vi "Frontend FPP_vdp_Ian_modified v3.0.vi"() -> ()   [LabVIEW 2016]
panel:
  in  "Gate 2":T1={"Gate Start"=0.0, "Gate Stop"=2.0, "Gate Step (linear only)"=1.0, "Gate Compliance"=0.0001, "Gate PComp"=0.0, "Range mode"=0, "Range"=6} {"Range" max=11 scale=0.0..11.0; "Range mode" items=["Auto", "Limited", "Fixed"]; "Gate PComp" format="%^.2e"; "Gate Compliance" format="%^.2e"; "Gate Step (linear only)" format="%^.4e"; "Gate Stop" format="%^.4e"; "Gate Start" format="%^.4e"}
  in  "Drain":T2={"Drain Start"=0.0, "Drain Stop"=2.0, "Drain Compliance"=0.0001, "Drain Step"=1.0, "Drain PComp"=0.0, "Range mode"=0, "Range"=6} {"Range" max=11 scale=0.0..11.0; "Range mode" items=["Auto", "Limited", "Fixed"]; "Drain PComp" format="%^.2e"; "Drain Step" format="%^.4e"; "Drain Compliance" format="%^.2e"; "Drain Stop" format="%^.4e"; "Drain Start" format="%^.4e"}
  in  "Gate":T3={"Gate Start"=0.0, "Gate Stop"=2.0, "Gate Step"=1.0, "Gate Compliance"=0.0001, "Gate PComp"=0.0, "Range mode"=0, "Range"=6} {"Range" max=11 scale=0.0..11.0; "Range mode" items=["Auto", "Limited", "Fixed"]; "Gate PComp" format="%^.2e"; "Gate Compliance" format="%^.2e"; "Gate Step" format="%^.4e"; "Gate Stop" format="%^.4e"; "Gate Start" format="%^.4e"}
  in  "Drain 2":T4={"Drain Start"=0.0, "Drain Stop"=2.0, "Drain Compliance"=0.0001, "Drain Step (linear only)"=1.0, "Drain PComp"=0.0, "Range mode"=0, "Range"=6} {"Range" max=11 scale=0.0..11.0; "Range mode" items=["Auto", "Limited", "Fixed"]; "Drain PComp" format="%^.2e"; "Drain Step (linear only)" format="%^.4e"; "Drain Compliance" format="%^.2e"; "Drain Stop" format="%^.4e"; "Drain Start" format="%^.4e"}
  in  "Timings":T5={"integration time"=0, "Short/Long integration time"=0.00064, "hold time (sec)"=0.0, "delay time (sec)"=0.0, "Step Time (0 disables)"=0.0, "sweep method"=0, "Pulse period"=0.005, "Base voltage"=0.0, "Pulse width"=0.0005} {"Pulse width" min=0.0005 max=0.1 step=0.0001 format="%.4f"; "Base voltage" format="%^.4e"; "Pulse period" min=0.005 max=1.0 step=0.0001 format="%.4f"; "sweep method" items=["Continuous", "Pulsed"]; "Step Time (0 disables)" format="%.2f"; "delay time (sec)" format="%.4f"; "hold time (sec)" format="%.4f"; "Short/Long integration time" format="%^.0e"; "integration time" scale=0.0..2.0}
  in  "Panel controls":T6={"Emergency Stop"=refnum, "OutputGraph Max"=1e-05, "Text/Graph (text=false)"=FALSE} {"OutputGraph Max" format="%.2e"}
  in  "Panel Controls":T7={"Emergency Stop"=refnum, "TransGraph Max"=1e-05, "Text/Graph (text=false)"=FALSE} {"TransGraph Max" format="%.2e"}
  in  "Tab Control":enum32{"Characteristics", "Other parameters"}(tab)
  in  "FPP - Source":u32(ring)=6 items=["SMU1  ", "SMU2  ", "SMU3  ", "SMU4  ", "SMU5  ", "SMU6  ", "VSU1  ", "VSU2  "]
  in  "FPP - Drain":u32(ring)=1 items=["SMU1  ", "SMU2  ", "SMU3  ", "SMU4  ", "SMU5  ", "SMU6  ", "VSU1  ", "VSU2  "]
  in  "FPP - Gate":u32(ring)=2 items=["SMU1  ", "SMU2  ", "SMU3  ", "SMU4  ", "SMU5  ", "SMU6  ", "VSU1  ", "VSU2  "]
  in  "FPP - Probe 1":u32(ring) items=["SMU1  ", "SMU2  ", "SMU3  ", "SMU4  ", "SMU5  ", "SMU6  ", "VSU1  ", "VSU2  "]
  in  "FPP - Probe 2":u32(ring)=3 items=["SMU1  ", "SMU2  ", "SMU3  ", "SMU4  ", "SMU5  ", "SMU6  ", "VSU1  ", "VSU2  "]
  in  "Van der Pauw":bool
  out "XY Graph 2":cluster{"Y data in":dbl[], "X data in":dbl[]}[](graph)
  in  "Integration time (long)":dbl=0.32 min=0.04 max=2.0 step=0.02 format="%.2f"
  in  "Integration time (short)":dbl=0.00064 min=8e-05 max=0.00192 step=8e-05 format="%^.0e"
  in  "Drain Range":u8(slide)=6 max=11 scale=0.0..11.0
  in  "Drain Range mode":u16(ring) items=["Auto", "Limited", "Fixed"]
  in  "Gate Range":u8(slide)=6 max=11 scale=0.0..11.0
  in  "Gate Range mode":u16(ring) items=["Auto", "Limited", "Fixed"]
  in  "Sampling mode":u32(slide) scale=0.0..4.0
  in  "Number of Samples":i32=500 min=0 step=1
  in  "Time":dbl=240.0 min=0.0 format="%.2f"
  in  "Drain":dbl=-10.0 min=-100.0 max=100.0 format="%.2f"
  in  "Gate":dbl=-60.0 min=-100.0 max=100.0 format="%.2f"
  in  "sweep method":u16(ring) items=["Continuous", "Pulsed"]
  out "Id":dbl format="%.2e"
  out "Ig":dbl format="%.2e"
  in  "Sweep Start":bool caption="Sweep start"
  in  "Interrupt run":bool
  in  "Running":bool=TRUE
  out "Path":path
  in  "integration time":u32(slide)=1 max=2 step=1 scale=0.0..2.0
  in  "sweep mode":u16(ring)=1 items=["Single", "Double"]
  in  "Transfer Start":bool
  in  "Output Start":bool
  in  "Drain: Step":dbl=-0.1 min=-100.0 max=100.0 format="%.2f"
  in  "Drain: Stop":dbl=-1.0 min=-100.0 max=100.0 format="%.2f"
  in  "Drain:Start":dbl=1.0 min=-100.0 max=100.0 format="%.2f"
  in  "Gate: Step":dbl min=-100.0 max=100.0 format="%.2f"
  in  "Gate: Stop":dbl min=-100.0 max=100.0 format="%.2f"
  in  "Gate: Start":dbl min=-100.0 max=100.0 format="%.2f"
  out "XY Graph":cluster{"Y data in":dbl[], "X data in":dbl[]}[](graph)
  in  "Drain: Compliance":dbl=0.001 min=1e-12 max=0.02 format="%.8f"
  in  "Gate: Compliance":dbl=0.001 min=1e-12 max=0.02 format="%.8f"
  in  "Drain: Step":dbl=-5.0 min=-100.0 max=100.0 format="%.2f"
  in  "Drain: Stop":dbl=-10.0 min=-100.0 max=100.0 format="%.2f"
  in  "Drain:Start":dbl=-5.0 min=-100.0 max=100.0 format="%.2f"
  in  "Gate: Step":dbl=-1.0 min=-100.0 max=100.0 format="%.2f"
  in  "Gate: Stop":dbl=-60.0 min=-100.0 max=100.0 format="%.2f"
  in  "Gate: Start":dbl=10.0 min=-100.0 max=100.0 format="%.2f"
  out "Vp_2":dbl format="%.2e"
  out "Vp_1":dbl format="%.2e"
  out "Delta V":dbl format="%.2e"
  out "Conductivity (S/cm)":dbl format="%.2e"
  in  "Thickness (m)":dbl=4e-08 min=1e-09 max=100.0 format="%.2e"
  in  "Hall Bar Channel Length  (L in m)":dbl=2e-05 format="%#_13g"
  in  "Hall Bar Channel Width (W in m)":dbl=4e-05 format="%#_13g"
  in  "Pulse width":dbl=0.0005 min=0.0005 max=0.1 step=0.0001 format="%.4f"
  in  "Base voltage":dbl min=-100.0 max=100.0 format="%.2f"
  in  "Pulse period":dbl=0.005 min=0.005 max=1.0 step=0.0001 format="%.4f"
  in  "Drain Power Compliance":dbl min=0.0 max=1.0 format="%.2f"
  in  "Gate Power\nCompliance":dbl min=0.0 max=1.0 format="%.2f"
  in  "OutputGraph Max":dbl=1e-05 format="%.2e"
  in  "TransGraph Max":dbl=1e-05 format="%.2e"
  in  "SPA Display":bool
  in  "Step delay /s":dbl min=0.0 max=1.0 format="%.2f"
  in  "hold time /s":dbl min=0.0 max=655.35 step=0.01 format="%.2f"
  in  "delay time /s":dbl min=0.0 max=65.535 step=0.0001 format="%.2f"
  in  "Decimal places in header":i8=1
  out "error out":errorcluster
  # "Transfer Characteristics"
  # "Stress Measurements"
  # "V"
  # "V"
  # "V"
  # "Gate"
  # "V"
  # "V"
  # "V"
  # "V"
  # "Drain"
  # "V"
  # "Output Characteristics"
  # "s"
  # "V"
  # "V"
  # "V"
  # "Gate"
  # "V"
  # "V"
  # "Drain"
  # "V"
  # "For Four Point Probe measurements ONLY!"
  # "A"
  # "A"
  # "Vp1"
  # "Vp2"
  # "Pulsed mode settings"
  # "NOTE - THIS OVERRIDES THE COMPLIANCE VALUES!"
  # "A"
  # "A"
  # "Enter max power in Watts (max 1W)"
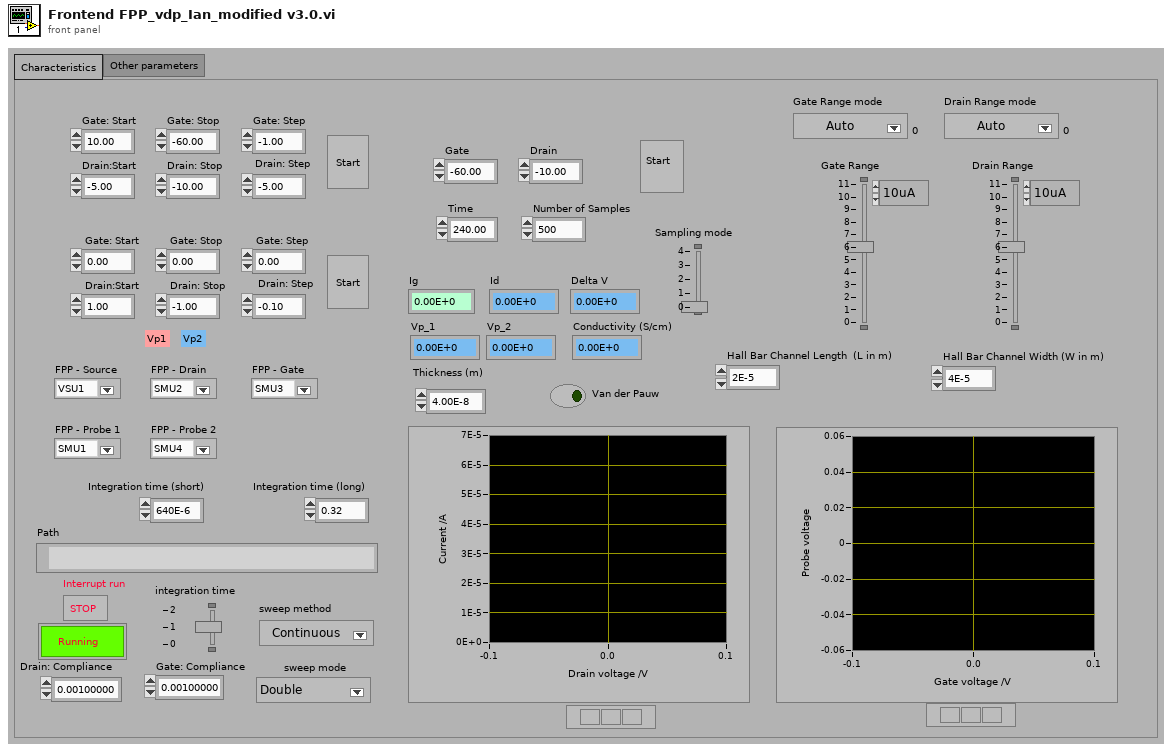
[diagram p1: front panel]
types:
  T1 = cluster{"Gate Start":dbl, "Gate Stop":dbl, "Gate Step (linear only)":dbl, "Gate Compliance":dbl, "Gate PComp":dbl, "Range mode":u16, "Range":u8}
  T2 = cluster{"Drain Start":dbl, "Drain Stop":dbl, "Drain Compliance":dbl, "Drain Step":dbl, "Drain PComp":dbl, "Range mode":u16, "Range":u8}
  T3 = cluster{"Gate Start":dbl, "Gate Stop":dbl, "Gate Step":dbl, "Gate Compliance":dbl, "Gate PComp":dbl, "Range mode":u16, "Range":u8}
  T4 = cluster{"Drain Start":dbl, "Drain Stop":dbl, "Drain Compliance":dbl, "Drain Step (linear only)":dbl, "Drain PComp":dbl, "Range mode":u16, "Range":u8}
  T5 = cluster{"integration time":u32, "Short/Long integration time":dbl, "hold time (sec)":dbl, "delay time (sec)":dbl, "Step Time (0 disables)":dbl, "sweep method":u16, "Pulse period":dbl, "Base voltage":dbl, "Pulse width":dbl}
  T6 = cluster{"Emergency Stop":refnum<vi>, "OutputGraph Max":dbl, "Text/Graph (text=false)":bool}
  T7 = cluster{"Emergency Stop":refnum<vi>, "TransGraph Max":dbl, "Text/Graph (text=false)":bool}
  T8 = cluster{"V2 Start":dbl, "V2 Step":dbl, "Number of points":i32}
  T9 = enum16{"open", "replace", "create", "open or create", "replace or create", "replace or create with confirmation"}
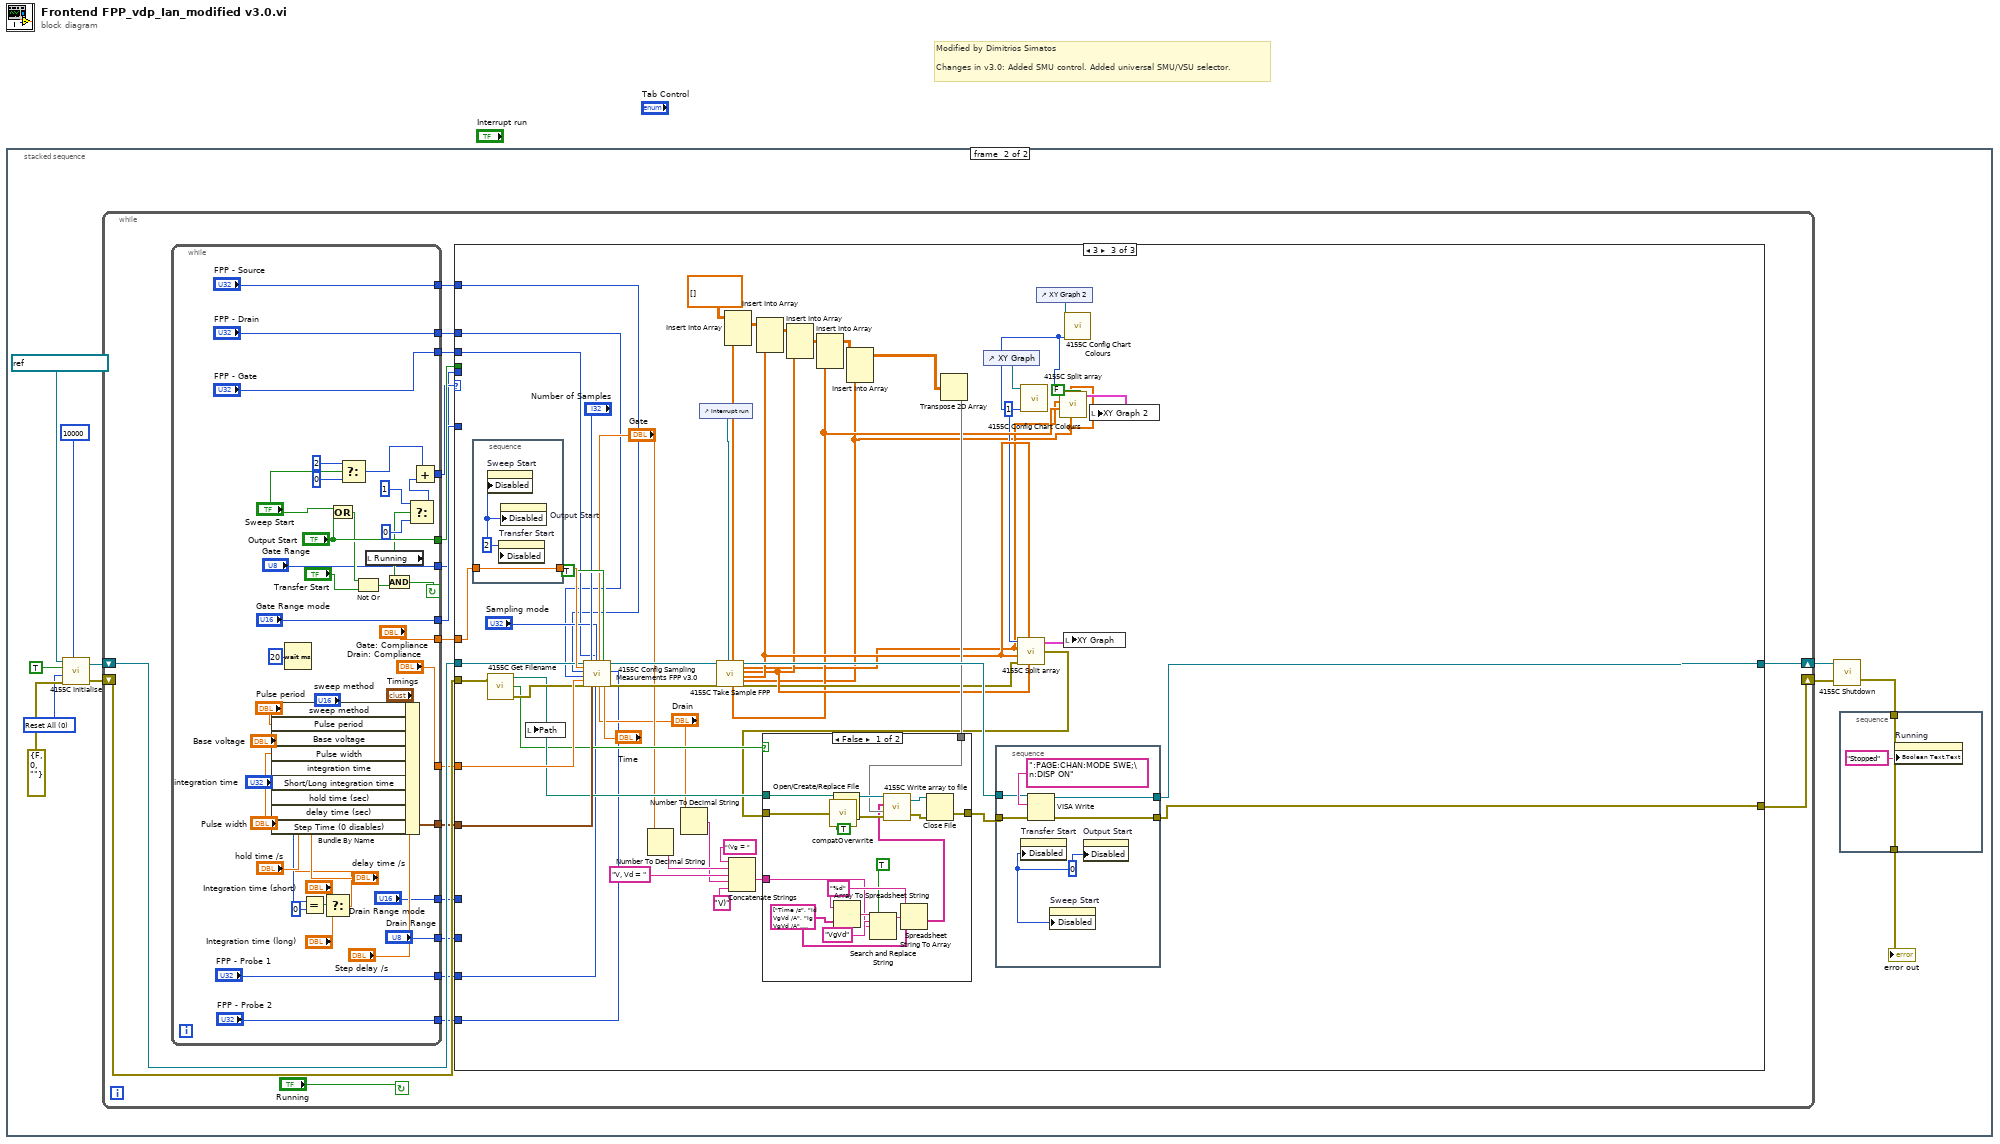
[diagram p0: block diagram]
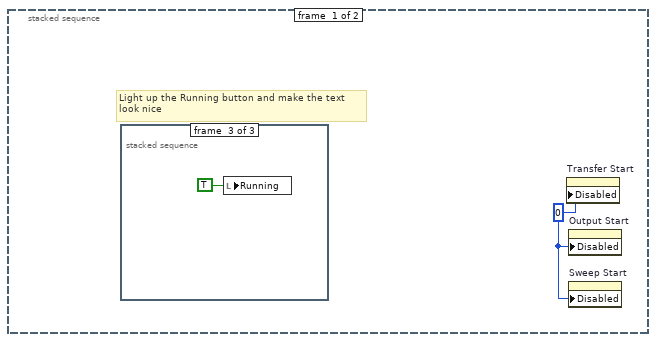
[diagram p2: hidden frame]
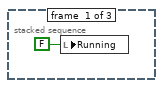
[diagram p3: hidden frame]
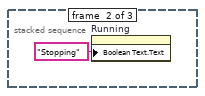
[diagram p4: hidden frame]
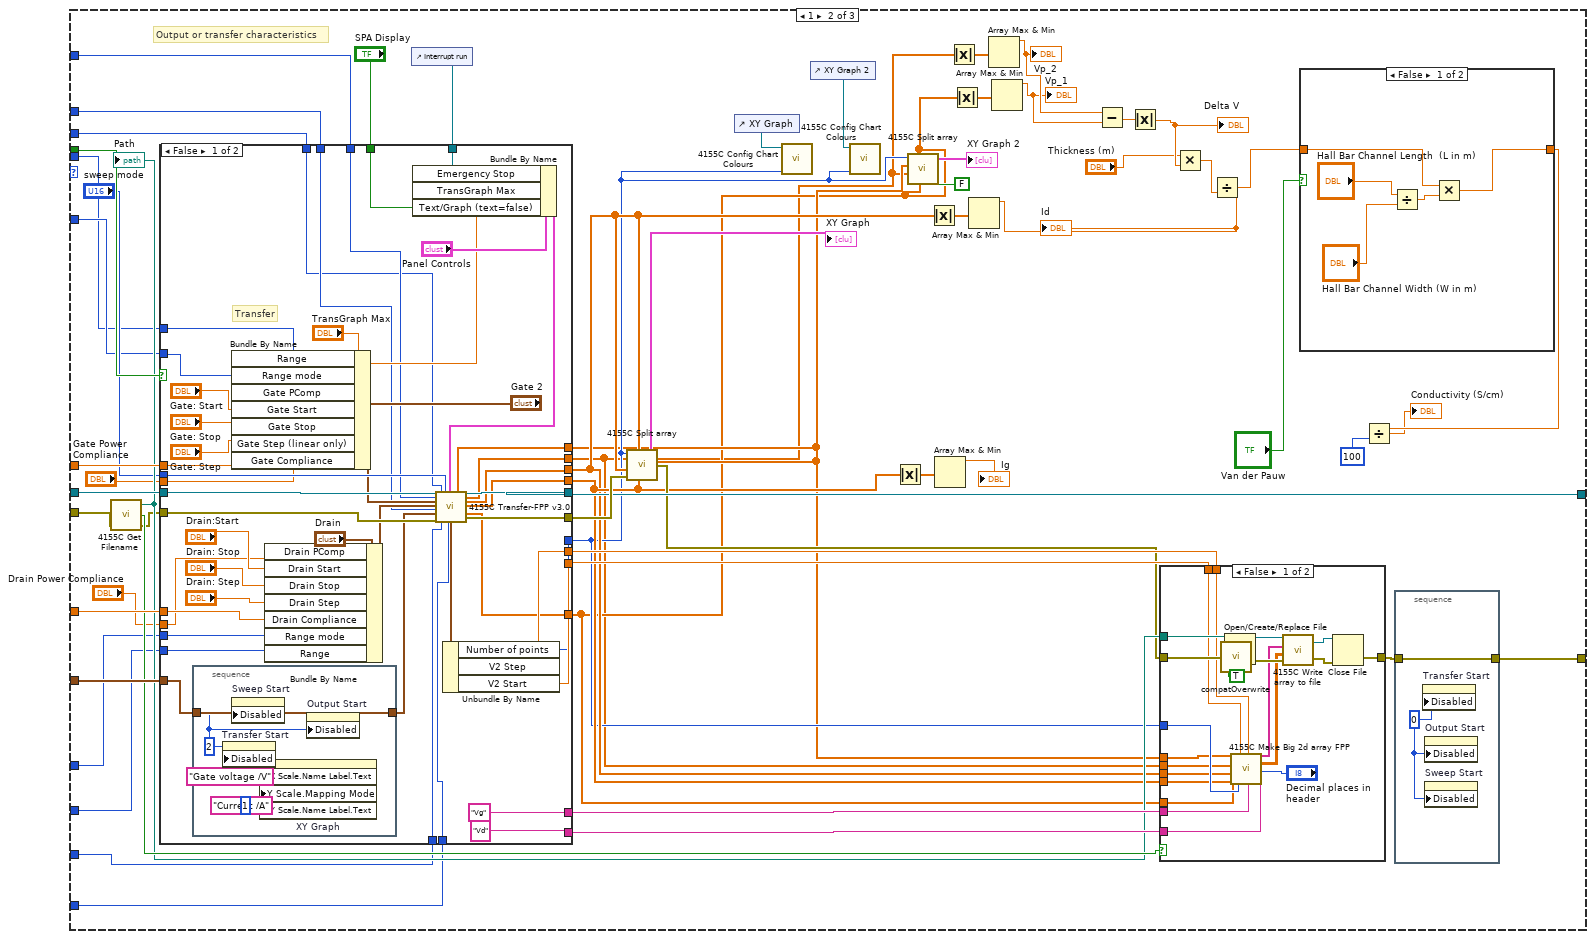
[diagram p6: hidden frame]
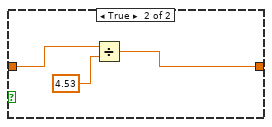
[diagram p7: hidden frame]
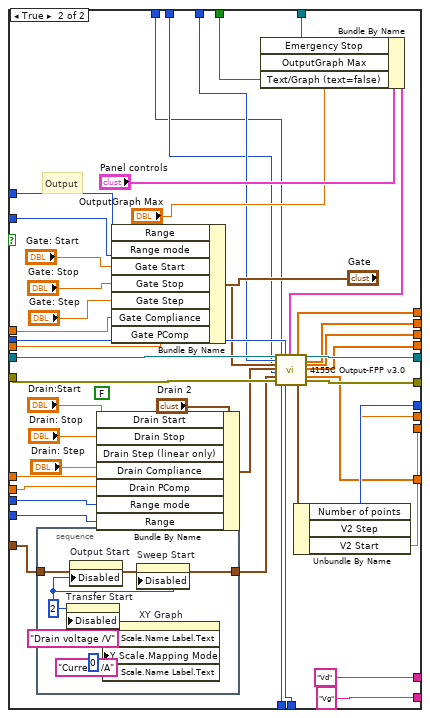
[diagram p9: hidden frame]
diagram:
  # "Modified by Dimitrios Simatos\n\nChanges in v3.0: Added SMU control. Added universal SMU/VSU selector."
  n1 = stacked-sequence {
    frame #0 {
      w1 = u8 0 ("Disabled")
      # "Light up the Running button and make the text\nlook nice"
      n2 = stacked-sequence {
        frame #0 {
          n3 = local write "Running"(FALSE ("Running")) -> ()
        }
        frame #1 {
          n4 = property on="Running" class="Bool (strict)"("Boolean Text.Text"="Stopping") -> ()  [unwired: 2 in, 2 out]
        }
        frame #2 {
          (unwired) FALSE ("Running")
          n5 = local write "Running"(TRUE ("Running")) -> ()
        }
      }
      n6 = property on="Transfer Start" class="Bool (strict)"("Disabled"=w1) -> ()  [unwired: 2 in, 2 out]
      n7 = property on="Output Start" class="Bool (strict)"("Disabled"=w1) -> ()  [unwired: 2 in, 2 out]
      n8 = property on="Sweep Start" class="Bool (strict)"("Disabled"=w1) -> ()  [unwired: 2 in, 2 out]
    }
    frame #1 {
      w11 = u16 0 items=["Reset All", "Partial reset"] ("Type of reset")
      n9 = call "4155C Initialise.vi"("VISA resource name in"=refnum<visa-resource-name> "GPIB0::14::INSTR", "Reset"=TRUE, "Type of reset"=w11, "error in (no error)"=errorcluster {"status"=FALSE, "code"=0, "source"=""}, "VISA Timeout Value"=u32 10000) -> ("VISA Resource Name out"=w10:refnum<visa-resource-name>, "error out"=w9:errorcluster)
      n10 = while {
        shift-left: w10 -> [w29]
        shift-right: [w31] -> w5
        shift-left: w9 -> [w30]
        shift-right: [w32] -> w6
        stop <- "Running" continue-if-true
        n11 = while {
          tunnel: ["Gate Range"] -> w21
          tunnel: ["Gate Range mode"] -> w22
          tunnel: ["Drain Range"] -> w23
          tunnel: ["Drain Range mode"] -> w24
          tunnel: ["Drain: Compliance"] -> w25
          tunnel: [w59] -> w26
          tunnel: ["Gate: Compliance"] -> w27
          tunnel: [w65] -> w28
          tunnel: ["Output Start"] -> w33
          tunnel: ["FPP - Probe 1"] -> w20
          tunnel: ["FPP - Probe 2"] -> w19
          tunnel: ["FPP - Gate"] -> w18
          tunnel: ["FPP - Drain"] -> w17
          tunnel: ["FPP - Source"] -> w16
          stop <- w74 continue-if-true
          n12 = Wait (ms)(milliseconds to wait=u32 20) -> ()  [unwired: 1 out]
          n13 = Equal?(x="integration time", y=u32 0) -> (x = y?=w56:bool)
          n14 = Select(t="Integration time (short)", s=w56, f="Integration time (long)") -> (s? t:f=w53:dbl)
          n15 = Bundle By Name(cluster="Timings", "sweep method"="sweep method", "Pulse period"="Pulse period", "Base voltage"="Base voltage", "Pulse width"="Pulse width", "integration time"="integration time", "Short/Long integration time"=w53, "hold time (sec)"="hold time /s", "delay time (sec)"="delay time /s", "Step Time (0 disables)"="Step delay /s") -> (w59:T5)
          n16 = Or(x="Sweep Start", y="Output Start") -> (x .or. y?=w71:bool)
          n17 = Select(t=i8 2, s="Sweep Start", f=i8 0) -> (s? t:f=w41:i8)
          n18 = Not Or(1:"Transfer Start", 2:w71) -> (0:w73:bool)
          n19 = local read "Running"() -> (w68:bool)
          n20 = And(x=w68, y=w73) -> (x .and. y?=w74:bool)
          n21 = Select(t=i8 1, s=w68, f=i8 0) -> (s? t:f=w64:i8)
          n22 = Add(x=w41, y=w64) -> (x+y=w65:i8)
        }
        n23 = case shown="3" w28 {
          tunnel: w33 -> [_ w137 _]
          tunnel: w26 -> [_ w136 w317]
          tunnel: w27 -> [_ w135 w325]
          tunnel: w25 -> [_ w134 w321]
          tunnel: [w77 w125 w323] -> w32
          tunnel: [w76 w128 w324] -> w31
          tunnel: w30 -> [w77 w119 w312]
          tunnel: w29 -> [w76 w127 w311]
          tunnel: w24 -> [_ w109 _]
          tunnel: w23 -> [_ w108 _]
          tunnel: w22 -> [_ w107 _]
          tunnel: w21 -> [_ w106 _]
          tunnel: w20 -> [_ w79 w277]
          tunnel: w19 -> [_ w78 w276]
          tunnel: w18 -> [_ w80 w275]
          tunnel: w17 -> [_ w81 w274]
          tunnel: w16 -> [_ w82 w273]
          frame 0, Default {
            # "Someone's deselected the running button so just shutdown..."
          }
          frame 1 {
            # "Output or transfer characteristics"
            n24 = call "4155C Get Filename.vi"("error in (no error)"=w119) -> ("error out"=w118:errorcluster, "cancelled"=w124:bool, "path"=w123:path)  [unwired: 2 in]
            "Path" <- w123
            n25 = control-ref of="Interrupt run"() -> (w120:refnum<vi>)
            n26 = case shown="False" w137 {
              tunnel: w127 -> [w202 w253]
              tunnel: w118 -> [w201 w252]
              tunnel: w136 -> [w205 w258]
              tunnel: w135 -> [w211 w265]
              tunnel: w134 -> [w216 w264]
              tunnel: "sweep mode" -> [w210 w263]
              tunnel: [w178 w231] -> w100
              tunnel: [w177 w230] -> w95
              tunnel: [w180 w229] -> w105
              tunnel: [w179 w228] -> w110
              tunnel: [w209 w262] -> w128
              tunnel: [w208 w261] -> w133
              tunnel: [w181 w234] -> w101
              tunnel: [w182 w233] -> w131
              tunnel: [w183 w232] -> w132
              tunnel: ["Vg" "Vd"] -> w130
              tunnel: ["Vd" "Vg"] -> w129
              tunnel: w120 -> [w199 w251]
              tunnel: "SPA Display" -> [w198 w249]
              tunnel: "Drain Power Compliance" -> [w194 w246]
              tunnel: "Gate Power\nCompliance" -> [w195 w245]
              tunnel: w109 -> [w186 w239]
              tunnel: w108 -> [w185 w238]
              tunnel: w107 -> [w187 w237]
              tunnel: w106 -> [w188 w236]
              tunnel: [w176 w227] -> w97
              tunnel: w82 -> [w175 w226]
              tunnel: w81 -> [w174 w225]
              tunnel: w80 -> [w173 w224]
              tunnel: w79 -> [w172 w223]
              tunnel: w78 -> [w171 w222]
              frame False {
                # "Transfer"
                n27 = stacked-sequence {
                  tunnel: w205 -> [w220]
                  tunnel: [w220] -> w193
                  frame #0 {
                    w218 = u8 2 ("Disabled")
                    n28 = property on="Transfer Start" class="Bool (strict)"("Disabled"=w218) -> ()  [unwired: 2 in, 2 out]
                    n29 = property on="Sweep Start" class="Bool (strict)"("Disabled"=w218) -> ()  [unwired: 2 in, 2 out]
                    n30 = property on="XY Graph" class="XYGraph (strict)"("X Scale.Name Label.Text"="Gate voltage /V", "Y Scale.Mapping Mode"=u8 1, "Y Scale.Name Label.Text"="Current /A") -> ()  [unwired: 2 in, 2 out]
                    n31 = property on="Output Start" class="Bool (strict)"("Disabled"=w218) -> ()  [unwired: 2 in, 2 out]
                  }
                }
                n32 = Bundle By Name(cluster="Gate 2", "Range"=w188, "Range mode"=w187, "Gate PComp"=w195, "Gate Start"="Gate: Start", "Gate Stop"="Gate: Stop", "Gate Step (linear only)"="Gate: Step", "Gate Compliance"=w211) -> (w189:T1)
                n33 = Bundle By Name(cluster="Drain", "Drain PComp"=w194, "Drain Start"="Drain:Start", "Drain Stop"="Drain: Stop", "Drain Step"="Drain: Step", "Drain Compliance"=w216, "Range mode"=w186, "Range"=w185) -> (w191:T2)
                n34 = Bundle By Name(cluster="Panel Controls", "Emergency Stop"=w199, "TransGraph Max"="TransGraph Max", "Text/Graph (text=false)"=w198) -> (w196:T7)
                n35 = call "4155C Transfer-FPP v3.0.vi"("VISA resource name in"=w202, "FPP - Source"=w175, "Gate"=w189, "Drain"=w191, "FPP - Drain"=w174, "Timings"=w193, "error in (no error)"=w201, "FPP - Gate"=w173, "FPP - Probe 1"=w172, "sweep mode"=w210, "FPP - Probe 2"=w171, "Panel Controls"=w196) -> ("VG"=w178:dbl[], "Outparams"=w184:T8, "VISA Resource Name out"=w209:refnum<visa-resource-name>, "Vprobe2"=w177:dbl[], "ID"=w180:dbl[], "IG"=w179:dbl[], "Vprobe1"=w176:dbl[], "error out"=w208:errorcluster)  [unwired: 8 in]
                n36 = Unbundle By Name(w184) -> ("Number of points"=w181:i32, "V2 Step"=w182:dbl, "V2 Start"=w183:dbl)
              }
              frame True {
                (unwired) FALSE ("Logarithmic")
                # "Output"
                n37 = stacked-sequence {
                  tunnel: w258 -> [w271]
                  tunnel: [w271] -> w244
                  frame #0 {
                    w269 = u8 2 ("Disabled")
                    n38 = property on="Transfer Start" class="Bool (strict)"("Disabled"=w269) -> ()  [unwired: 2 in, 2 out]
                    n39 = property on="Output Start" class="Bool (strict)"("Disabled"=w269) -> ()  [unwired: 2 in, 2 out]
                    n40 = property on="XY Graph" class="XYGraph (strict)"("X Scale.Name Label.Text"="Drain voltage /V", "Y Scale.Mapping Mode"=u8 0, "Y Scale.Name Label.Text"="Current /A") -> ()  [unwired: 2 in, 2 out]
                    n41 = property on="Sweep Start" class="Bool (strict)"("Disabled"=w269) -> ()  [unwired: 2 in, 2 out]
                  }
                }
                n42 = Bundle By Name(cluster="Drain 2", "Drain Start"="Drain:Start", "Drain Stop"="Drain: Stop", "Drain Step (linear only)"="Drain: Step", "Drain Compliance"=w264, "Drain PComp"=w246, "Range mode"=w239, "Range"=w238) -> (w242:T4)
                n43 = Bundle By Name(cluster="Gate", "Range"=w236, "Range mode"=w237, "Gate Start"="Gate: Start", "Gate Stop"="Gate: Stop", "Gate Step"="Gate: Step", "Gate Compliance"=w265, "Gate PComp"=w245) -> (w240:T3)
                n44 = Bundle By Name(cluster="Panel controls", "Emergency Stop"=w251, "OutputGraph Max"="OutputGraph Max", "Text/Graph (text=false)"=w249) -> (w247:T6)
                n45 = call "4155C Output-FPP v3.0.vi"("VISA resource name in"=w253, "FPP - Source"=w226, "Gate"=w240, "Drain"=w242, "FPP - Drain"=w225, "Timings"=w244, "error in (no error)"=w252, "FPP - Gate"=w224, "FPP - Probe 1"=w223, "sweep mode"=w263, "FPP - Probe 2"=w222, "Panel controls"=w247) -> ("VD"=w231:dbl[], "Outparams"=w235:T8, "VISA Resource Name out"=w262:refnum<visa-resource-name>, "Vprobe2"=w230:dbl[], "ID"=w229:dbl[], "IG"=w228:dbl[], "Vprobe1"=w227:dbl[], "error out"=w261:errorcluster)  [unwired: 8 in]
                n46 = Unbundle By Name(w235) -> ("Number of points"=w234:i32, "V2 Step"=w233:dbl, "V2 Start"=w232:dbl)
              }
            }
            n47 = call "4155C Split array.vi"("Number of VAR2 steps"=w101, "Y2 data in"=w105, "X data in"=w100, "Y1 data in"=w105, "Y3 data in"=w110, "error in (no error)"=w133) -> ("Array of clusters"=→"XY Graph":cluster{"Y data in":dbl[], "X data in":dbl[]}[], "error out"=w117:errorcluster)  [unwired: 1 in]
            n48 = control-ref of="XY Graph"() -> (w121:refnum<vi>)
            n49 = call "4155C Config Chart Colours.vi"("Numeric"=w101, "XY Graph 2"=w121) -> ()  [unwired: 6 in]
            n50 = control-ref of="XY Graph 2"() -> (w103:refnum<vi>)
            n51 = call "4155C Config Chart Colours.vi"("Numeric"=w101, "XY Graph 2"=w103) -> ()  [unwired: 6 in]
            n52 = Absolute Value(x=w110) -> (abs(x)=w112:dbl[])
            n53 = call "4155C Split array.vi"("Number of VAR2 steps"=w101, "Y2 data in"=w97, "X data in"=w100, "Y1 data in"=w95, "Y3 data in"=w97, "Absolute val?"=FALSE) -> ("Array of clusters"=→"XY Graph 2":cluster{"Y data in":dbl[], "X data in":dbl[]}[])  [unwired: 1 in, 1 out]
            n54 = Absolute Value(x=w105) -> (abs(x)=w111:dbl[])
            n55 = Array Max & Min(array=w112) -> (max value=→"Ig":dbl)  [unwired: 3 out]
            n56 = Absolute Value(x=w95) -> (abs(x)=w96:dbl[])
            n57 = Absolute Value(x=w97) -> (abs(x)=w98:dbl[])
            n58 = Array Max & Min(array=w111) -> (max value=w86:dbl)  [unwired: 3 out]
            "Id" <- w86
            n59 = Array Max & Min(array=w96) -> (max value=w94:dbl)  [unwired: 3 out]
            "Vp_2" <- w94
            n60 = Array Max & Min(array=w98) -> (max value=w93:dbl)  [unwired: 3 out]
            "Vp_1" <- w93
            n61 = Subtract(x=w94, y=w93) -> (x-y=w92:dbl)
            n62 = Absolute Value(x=w92) -> (abs(x)=w91:dbl)
            "Delta V" <- w91
            n63 = case shown="False" w124 {
              tunnel: w117 -> [w168 w170]
              tunnel: [w163 w170] -> w126
              tunnel: w123 -> [w167 _]
              tunnel: w101 -> [w161 _]
              tunnel: w105 -> [w151 _]
              tunnel: w100 -> [w153 _]
              tunnel: w95 -> [w152 _]
              tunnel: w110 -> [w150 _]
              tunnel: w132 -> [w155 _]
              tunnel: w131 -> [w156 _]
              tunnel: w130 -> [w160 _]
              tunnel: w129 -> [w159 _]
              tunnel: w97 -> [w149 _]
              frame False {
                n64 = call <vilib>:"compatOverwrite.vi"("overwrite (F)"=TRUE) -> ("overwrite?"=w148:T9)
                n65 = Open/Create/Replace File(file path (use dialog)=w167, error in=w168, operation (0:open)=w148) -> (refnum out=w165:refnum<file>, error out=w166:errorcluster)  [unwired: 3 in, 1 out]
                n66 = call "4155C Make Big 2d array FPP.vi"("1D Var1"=w153, "1d ID"=w151, "1d Vp2"=w152, "1d IG"=w150, "1d Vp1"=w149, "VAR2 START"=w155, "Number of VAR2 steps"=w161, "VAR2 STEP"=w156, "VAR1 Name"=w160, "Decimal places in header"="Decimal places in header", "VAR2 Name"=w159) -> ("Header array"=w157:string[], "Data array"=w158:dbl[][])  [unwired: 15 in]
                n67 = call "4155C Write array to file.vi"("Byte Stream File Refnum"=w165, "Header"=w157, "Data Array"=w158, "error in (no error)"=w166) -> ("dup refnum"=w162:refnum<file>, "error out"=w164:errorcluster)  [unwired: 1 in]
                n68 = Close File(refnum=w162, error in=w164) -> (error out=w163:errorcluster)  [unwired: 1 out]
              }
              frame True {
              }
            }
            n69 = Multiply(x="Thickness (m)", y=w91) -> (x*y=w87:dbl)
            n70 = Divide(x=w86, y=w87) -> (x/y=w88:dbl)
            n71 = case shown="False" "Van der Pauw" {
              tunnel: [w140 w144] -> w85
              tunnel: w88 -> [w141 w145]
              frame False {
                n72 = Divide(x="Hall Bar Channel Length  (L in m)", y="Hall Bar Channel Width (W in m)") -> (x/y=w142:dbl)
                n73 = Multiply(x=w141, y=w142) -> (x*y=w140:dbl)
              }
              frame True {
                n74 = Divide(x=w145, y=4.53) -> (x/y=w144:dbl)
              }
            }
            n75 = Divide(x=w85, y=100) -> (x/y=→"Conductivity (S/cm)":dbl)
            n76 = stacked-sequence {
              tunnel: w126 -> [w147]
              tunnel: [w147] -> w125
              frame #0 {
                w146 = u8 0 ("Disabled")
                n77 = property on="Transfer Start" class="Bool (strict)"("Disabled"=w146) -> ()  [unwired: 2 in, 2 out]
                n78 = property on="Output Start" class="Bool (strict)"("Disabled"=w146) -> ()  [unwired: 2 in, 2 out]
                n79 = property on="Sweep Start" class="Bool (strict)"("Disabled"=w146) -> ()  [unwired: 2 in, 2 out]
              }
            }
          }
          frame 3 {
            w281 = 1 ("Numeric")
            n80 = stacked-sequence {
              tunnel: w325 -> [w352]
              tunnel: [w352] -> w322
              frame #0 {
                w351 = u8 2 ("Disabled")
                n81 = property on="Sweep Start" class="Bool (strict)"("Disabled"=w351) -> ()  [unwired: 2 in, 2 out]
                n82 = property on="Transfer Start" class="Bool (strict)"("Disabled"=w351) -> ()  [unwired: 2 in, 2 out]
                n83 = property on="Output Start" class="Bool (strict)"("Disabled"=w351) -> ()  [unwired: 2 in, 2 out]
              }
            }
            n84 = call "4155C Get Filename.vi"("error in (no error)"=w312) -> ("error out"=w310:errorcluster, "cancelled"=w301:bool, "path"=w302:path)  [unwired: 2 in]
            n85 = local write "Path"(w302) -> ()
            n86 = call "4155C Config Sampling Measurements FPP v3.0.vi"("VISA session"=w311, "Gate Compliance"=w322, "FPP - Source"=w273, "FPP - Drain"=w274, "Drain Compliance"=w321, "error in (no error)"=w310, "Num Points"="Number of Samples", "Timings"=w317, "FPP - Gate"=w275, "FPP - Probe 1"=w277, "Vg"="Gate", "Vd"="Drain", "Display on/off"=TRUE, "Sample time"="Time", "Sampling mode"="Sampling mode", "FPP - Probe 2"=w276) -> ("dup VISA resource name"=w318:refnum<visa-resource-name>, "error out"=w319:errorcluster)  [unwired: 2 in]
            n87 = Number To Decimal String(number="Gate") -> (decimal integer string=w299:string)  [unwired: 1 in]
            n88 = Number To Decimal String(number="Drain") -> (decimal integer string=w297:string)  [unwired: 1 in]
            n89 = control-ref of="Interrupt run"() -> (w313:refnum<vi>)
            n90 = call "4155C Take Sample FPP.vi"("VISA resource name in"=w318, "error in (no error)"=w319, "Emergency Stop"=w313) -> ("Time"=w279:dbl[], "Vp1"=w283:dbl[], "VISA Resource Name out"=w320:refnum<visa-resource-name>, "Ig"=w291:dbl[], "Id"=w292:dbl[], "Vp2"=w278:dbl[], "error out"=w290:errorcluster)  [unwired: 10 in]
            n91 = Insert Into Array(array=dbl[][] [] ("Input Array"), new element=w279) -> (w309:dbl[][])  [unwired: 2 in]
            n92 = Concatenate Strings("(Vg = " ("Substring"), w299, "V, Vd = " ("Substring"), w297, "V)" ("Substring")) -> (w295:string)
            n93 = Insert Into Array(array=w309, new element=w292) -> (w308:dbl[][])  [unwired: 2 in]
            n94 = Insert Into Array(array=w308, new element=w291) -> (w307:dbl[][])  [unwired: 2 in]
            n95 = Insert Into Array(array=w307, new element=w283) -> (w305:dbl[][])  [unwired: 2 in]
            n96 = Insert Into Array(array=w305, new element=w278) -> (w285:dbl[][])  [unwired: 2 in]
            n97 = Transpose 2D Array(2D array=w285) -> (transposed array=w303:dbl[][])
            n98 = control-ref of="XY Graph"() -> (w294:refnum<vi>)
            n99 = call "4155C Split array.vi"("Number of VAR2 steps"=w281, "Y2 data in"=w292, "X data in"=w279, "Y1 data in"=w292, "Y3 data in"=w291, "error in (no error)"=w290) -> ("Array of clusters"=w293:cluster{"Y data in":dbl[], "X data in":dbl[]}[], "error out"=w289:errorcluster)  [unwired: 1 in]
            n100 = case shown="False" w301 {
              tunnel: w289 -> [w342 w344]
              tunnel: [w337 w344] -> w304
              tunnel: w302 -> [w341 _]
              tunnel: w303 -> [w335 _]
              tunnel: w295 -> [w327 _]
              frame False {
                w328 = string[] ["Time /s", "Id VgVd /A", "Ig VgVd /A", "Vp1 VgVd /V", "Vp2 VgVd /V"] ("Header")
                w332 = "%d" ("format string")
                n101 = call <vilib>:"compatOverwrite.vi"("overwrite (F)"=TRUE) -> ("overwrite?"=w326:T9)
                n102 = Open/Create/Replace File(file path (use dialog)=w341, error in=w342, operation (0:open)=w326) -> (refnum out=w339:refnum<file>, error out=w340:errorcluster)  [unwired: 3 in, 1 out]
                n103 = Array To Spreadsheet String(array=w328, 3:w332) -> (spreadsheet string=w334:string)  [unwired: 1 in]
                n104 = Search and Replace String(replace all?=TRUE ("replace all? (F)"), input string=w334, search string="VgVd", replace string=w327) -> (result string=w330:string)  [unwired: 4 in, 3 out]
                n105 = Spreadsheet String To Array(format string=w332, spreadsheet string=w330, array type (2D Dbl)=w328) -> (array=w329:string[])  [unwired: 1 in]
                n106 = call "4155C Write array to file.vi"("Byte Stream File Refnum"=w339, "Header"=w329, "Data Array"=w335, "error in (no error)"=w340) -> ("dup refnum"=w336:refnum<file>, "error out"=w338:errorcluster)  [unwired: 1 in]
                n107 = Close File(refnum=w336, error in=w338) -> (error out=w337:errorcluster)  [unwired: 1 out]
              }
              frame True {
              }
            }
            n108 = stacked-sequence {
              tunnel: [w347] -> w324
              tunnel: [w346] -> w323
              tunnel: w320 -> [w349]
              tunnel: w304 -> [w348]
              frame #0 {
                w345 = u8 0 ("Disabled")
                n109 = property on="Transfer Start" class="Bool (strict)"("Disabled"=w345) -> ()  [unwired: 2 in, 2 out]
                n110 = VISA Write(VISA resource name=w349, write buffer=":PAGE:CHAN:MODE SWE;\n:DISP ON" ("write buffer (\"\")"), error in (no error)=w348) -> (VISA resource name out=w347:refnum<visa-resource-name>, error out=w346:errorcluster)  [unwired: 1 out]
                n111 = property on="Sweep Start" class="Bool (strict)"("Disabled"=w345) -> ()  [unwired: 2 in, 2 out]
                n112 = property on="Output Start" class="Bool (strict)"("Disabled"=w345) -> ()  [unwired: 2 in, 2 out]
              }
            }
            n113 = call "4155C Config Chart Colours.vi"("Numeric"=w281, "XY Graph 2"=w294) -> ()  [unwired: 6 in]
            n114 = control-ref of="XY Graph 2"() -> (w284:refnum<vi>)
            n115 = call "4155C Split array.vi"("Number of VAR2 steps"=w281, "Y2 data in"=w278, "X data in"=w279, "Y1 data in"=w283, "Y3 data in"=w278, "Absolute val?"=FALSE) -> ("Array of clusters"=w282:cluster{"Y data in":dbl[], "X data in":dbl[]}[])  [unwired: 1 in, 1 out]
            n116 = local write "XY Graph"(w293) -> ()
            n117 = call "4155C Config Chart Colours.vi"("Numeric"=w281, "XY Graph 2"=w284) -> ()  [unwired: 6 in]
            n118 = local write "XY Graph 2"(w282) -> ()
          }
        }
      }
      n119 = call "4155C Shutdown.vi"("VISA resource name in"=w5, "error in (no error)"=w6) -> ("error out"=w8:errorcluster)  [unwired: 4 in]
      n120 = stacked-sequence {
        tunnel: w8 -> [w354]
        tunnel: [w354] -> w7
        frame #0 {
          n121 = property on="Running" class="Bool (strict)"("Boolean Text.Text"="Stopped") -> ()  [unwired: 2 in, 2 out]
        }
      }
      "error out" <- w7
    }
  }
